vi "to string.vi"(8 "error in":errorcluster, 11 "Special Test configuration":refnum<class "Special Test configuration.lvclass">) -> (0 "error out":errorcluster, 1 "data":string, 2 "version":string, 3 "Special Test configuration out":refnum<class "Special Test configuration.lvclass">)   [LabVIEW 2025, in "Special Test.lvlib" / "Special Test configuration.lvclass"]
doc: "Provides an interface for saving a module configuration to a file or other serialized data source. It is recommended that all children of this class store data in two sets--data required for its own initialization, and any data required for parent initialization--and that each implementation uses the <b>Call Parent Method</b> primitive to serialize parent information.Copyright 2017 National Instruments Corporation\n\nLicensed under the Apache License, Version 2.0 (the \"License\"); you may not use this file except in compliance with the License. You may obtain a copy of the License at http://www.apache.org/licenses/LICENSE-2.0\nUnless required by applicable law or agreed to in writing, software distributed under the License is distributed on an \"AS IS\" BASIS, WITHOUT WARRANTIES OR CONDITIONS OF ANY KIND, either express or implied. See the License for the specific language governing permissions and limitations under the License."
uses:
  Special Test configuration.lvclass
  Special Test configuration.lvclass/Special Test configuration.ctl
  Users/Public/Documents/Sandia National Labs/TSS Plugin/CEF.lvlibp/serializable configuration/CEF_serializable configuration.lvclass
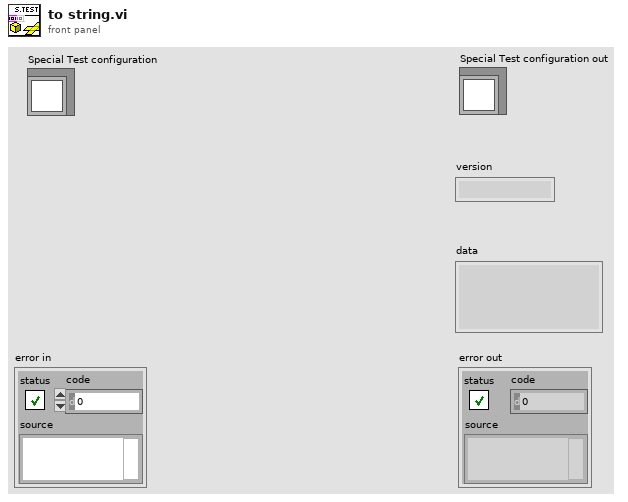
[diagram p1: front panel]
types:
  T1 = typedef "Special Test.lvlib/Special Test configuration.lvclass/Test Info.ctl" = cluster{"General":cluster{"Location":string, "Operator":string}, "Doc":cluster{"Shorthand Test Name":string, "MRS Code":string, "P6 Test Activity Name":string, "Test Plan":string, "Wiring Diagram":string}, "Test Setup":cluster{"Series":string, "Test Code":string, "Test Group":string, "Config Type":string}, "Run":cluster{"Temperature":string, "Voltage":string, "Attempt":u32, "Test Run":string, "Pre-Test Notes":string, "Source Code":string, "During Environment":string, "Enable Dropouts":bool}}
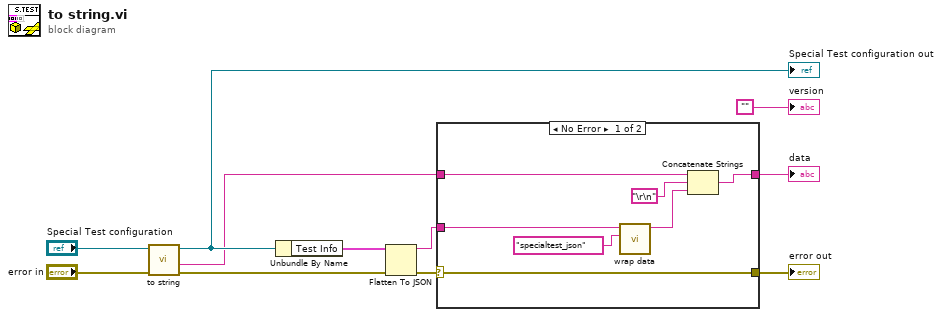
[diagram p0: block diagram]
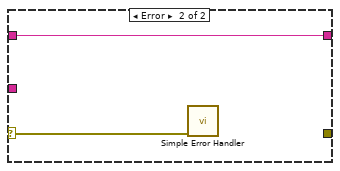
[diagram p2: hidden frame]
diagram:
  n1 = call-parent "to string.vi"("error in"="error in", "CEF_Configuration in"="Special Test configuration") -> ("error out"=w7:errorcluster, "data"=w3:string, "CEF_Configuration out"=w9:refnum<class "Special Test configuration.lvclass">)  [unwired: 6 in, 1 out]
  "Special Test configuration out" <- w9
  n2 = Unbundle By Name(w9) -> ("Test Info"=w8:T1)
  n3 = Flatten To JSON(anything=w8, error in (no error)=w7) -> (JSON string=w4:string, 11:w6:errorcluster)  [unwired: 1 in]
  n4 = case shown="No Error" w6 {
    selector: w6 -> [w18 w20]
    tunnel: [w18 _] -> w5
    tunnel: w4 -> [w15 _]
    tunnel: w3 -> [w14 w19]
    tunnel: [w12 w19] -> w2
    frame No Error {
      n5 = call "wrap data.vi"("identifier"="specialtest_json" ("additional identifier"), "data to wrap"=w15) -> ("wrapped data"=w17:string)  [unwired: 9 in]
      n6 = Concatenate Strings(w14, "\r\n", w17) -> (w12:string)
    }
    frame Error {
      n7 = call <vilib>:"Simple Error Handler.vi"("error in (no error)"=w20) -> ()  [unwired: 4 in, 5 out]
    }
  }
  "error out" <- w5
  "data" <- w2
  "version" <- ""
